vi "Set Property.vi"(0 "Refnum":refnum<vi>, 5 "Colors":refnum<vi>, 7 "Property":T1 {"Mech.Action" items=["Switch when Pressed", "Switch when Released", "Switch until Released", "Latch when Pressed", "Latch when Released", "Latch until Released"]; "Type" items=["Numeric", "Spin Control", "Vertical Slide", "Horizontal Slide", "Push Button", "Rocker", "Vert Rocker", "Horizontal Toggle Switch", "Vertical Toggle Switch", "Slide Switch", "Vertical Slide Switch", "OK Button", "Square Push Button", "Round Push Button", "Vertical Slide Switch2", "Square Push Button2", "Round Push Button2", "Horizontal Slide Switch2", "Round LED", "Square LED"]}, 11 "error in (no error)":errorcluster) -> (15 "error out":errorcluster)   [LabVIEW 2011]
uses:
  Default.ctl
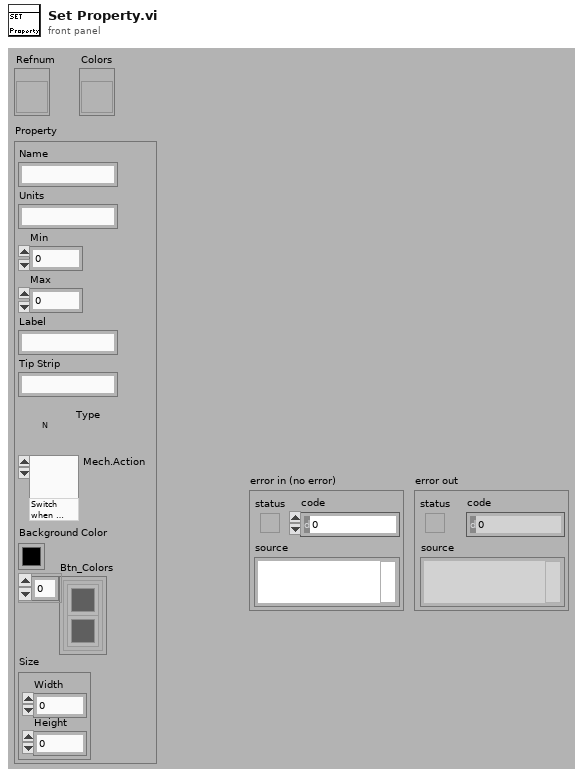
[diagram p1: front panel]
types:
  T1 = typedef "Default.ctl" = cluster{"Name":string, "Units":string, "Min":dbl, "Max":dbl, "Label":string, "Tip Strip":string, "Background Color":u32, "Type":i32, "Mech.Action":u16, "Btn_Colors ":cluster{"FG":u32, "BG":u32}[], "Size":cluster{"Width":u32, "Height":u32}}
  T2 = typedef "LVPositionTypeDef.ctl" = cluster{"Left":i32, "Top":i32}
  T3 = enum8{"Enabled", "Disabled", "Disabled and Grayed Out"}
  T4 = cluster{"Colors [4][0]":cluster{"FG":u32, "BG":u32}, "Colors [4][1]":cluster{"FG":u32, "BG":u32}, "Colors [4][2]":cluster{"FG":u32, "BG":u32}, "Colors [4][3]":cluster{"FG":u32, "BG":u32}}
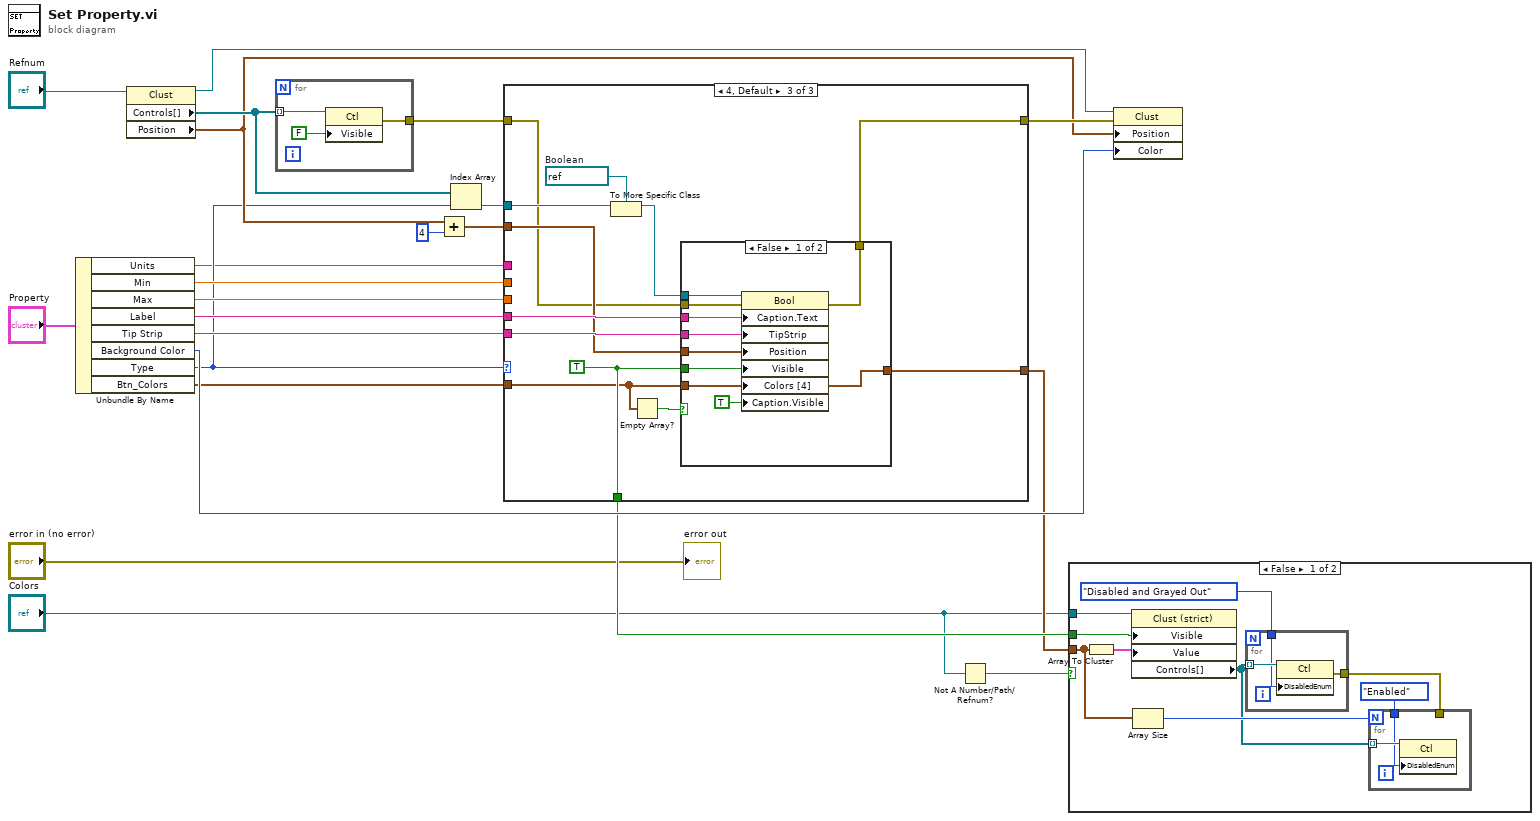
[diagram p0: block diagram]
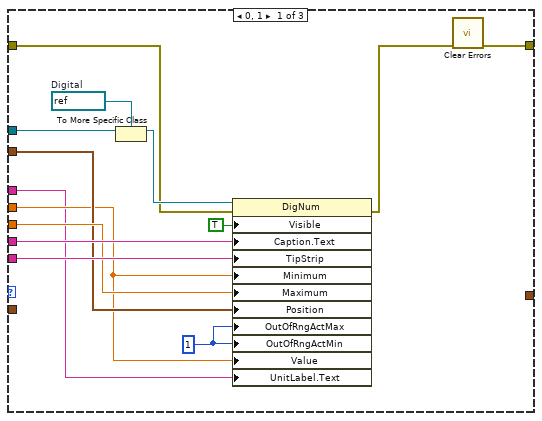
[diagram p3: hidden frame]
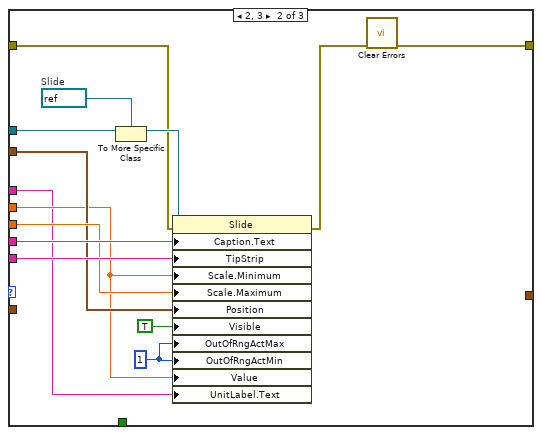
[diagram p4: hidden frame]
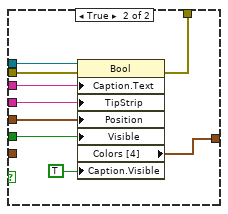
[diagram p5: hidden frame]
diagram:
  n1 = Unbundle By Name("Property") -> ("Units"=w2:string, "Min"=w22:dbl, "Max"=w21:dbl, "Label"=w20:string, "Tip Strip"=w19:string, "Background Color"=w10:u32, "Type"=w9:i32, "Btn_Colors"=w7:cluster{"FG":u32, "BG":u32}[])
  n2 = property class="Clust"(reference="Refnum") -> (reference out=w12:refnum<vi>, "Controls[]"=w17:refnum<vi>[], "Position"=w11:T2)  [unwired: 1 in, 1 out]
  n3 = for {
    tunnel: w17 -> [w26] mode=indexing
    tunnel: [w24] -> w14
    n4 = property class="Ctl"(reference=w26, "Visible"=FALSE) -> (error out=w24:errorcluster)  [unwired: 1 in, 1 out]
  }
  n5 = Add(x=w11, y=4) -> (x+y=w15:T2)
  n6 = Index Array(array=w17, index=w9) -> (element=w16:refnum<vi>)
  n7 = case shown="4, Default" w9 {
    tunnel: w2 -> [w27 w42 _]
    tunnel: w22 -> [w30 w43 _]
    tunnel: w21 -> [w36 w51 _]
    tunnel: w20 -> [w40 w54 w65]
    tunnel: w19 -> [w37 w52 w62]
    tunnel: w16 -> [w35 w50 w66]
    tunnel: w15 -> [w34 w47 w61]
    tunnel: w14 -> [w33 w46 w60]
    tunnel: [w29 w41 w59] -> w13
    tunnel: [_ _ w58] -> w8
    tunnel: w7 -> [_ _ w57]
    tunnel: [_ _ w55] -> w6
    frame 0, 1 {
      w31 = u8 1 ("Response to Value Outside Limits:Maximum")
      w38 = refnum<vi> refnum  # Digital
      n8 = To More Specific Class(target class=w38, reference=w35) -> (specific class reference=w39:refnum<vi>)  [unwired: 1 in, 1 out]
      n9 = property class="DigNum"(reference=w39, error in=w33, "Visible"=TRUE, "Caption.Text"=w40, "TipStrip"=w37, "Minimum"=w30, "Maximum"=w36, "Position"=w34, "OutOfRngActMax"=w31, "OutOfRngActMin"=w31, "Value"=w30, "UnitLabel.Text"=w27) -> (error out=w32:errorcluster)  [unwired: 1 out]
      n10 = call <vilib>:"Clear Errors.vi"("error in (no error)"=w32) -> ("error out"=w29:errorcluster)  [unwired: 6 in]
    }
    frame 2, 3 {
      w44 = u8 1 ("Response to Value Outside Limits:Maximum")
      w49 = refnum<vi> refnum  # Slide
      n11 = To More Specific Class(target class=w49, reference=w50) -> (specific class reference=w53:refnum<vi>)  [unwired: 1 in, 1 out]
      n12 = property class="Slide"(reference=w53, error in=w46, "Caption.Text"=w54, "TipStrip"=w52, "Scale.Minimum"=w43, "Scale.Maximum"=w51, "Position"=w47, "Visible"=TRUE, "OutOfRngActMax"=w44, "OutOfRngActMin"=w44, "Value"=w43, "UnitLabel.Text"=w42) -> (error out=w45:errorcluster)  [unwired: 1 out]
      n13 = call <vilib>:"Clear Errors.vi"("error in (no error)"=w45) -> ("error out"=w41:errorcluster)  [unwired: 6 in]
    }
    frame 4, Default {
      w58 = TRUE ("Visible")
      w63 = refnum<vi> refnum  # Boolean
      n14 = To More Specific Class(target class=w63, reference=w66) -> (specific class reference=w64:refnum<vi>)  [unwired: 1 in, 1 out]
      n15 = Empty Array?(array=w57) -> (empty?=w56:bool)
      n16 = case shown="False" w56 {
        tunnel: w65 -> [w75 w84]
        tunnel: w64 -> [w74 w83]
        tunnel: w62 -> [w73 w82]
        tunnel: w61 -> [w72 w81]
        tunnel: w60 -> [w71 w80]
        tunnel: [w70 w79] -> w59
        tunnel: w58 -> [w69 w78]
        tunnel: w57 -> [w68 _]
        tunnel: [w68 w77] -> w55
        frame False {
          n17 = property class="Bool"(reference=w74, error in=w71, "Caption.Text"=w75, "TipStrip"=w73, "Position"=w72, "Visible"=w69, "Colors [4]"=w68, "Caption.Visible"=TRUE) -> (error out=w70:errorcluster)  [unwired: 1 out]
        }
        frame True {
          n18 = property class="Bool"(reference=w83, error in=w80, "Caption.Text"=w84, "TipStrip"=w82, "Position"=w81, "Visible"=w78, "Caption.Visible"=TRUE) -> (error out=w79:errorcluster, "Colors [4]"=w77:cluster{u32, u32}[])  [unwired: 1 out]
        }
      }
    }
  }
  n19 = Not A Number/Path/Refnum?(number/path/refnum="Colors") -> (NaN/Path/Refnum?=w4:bool)
  n20 = case shown="False" w4 {
    tunnel: w8 -> [w93 _]
    tunnel: w6 -> [w90 _]
    tunnel: "Colors" -> [w92 _]
    frame False {
      n21 = Array To Cluster(array=w90) -> (cluster=w91:T4)
      n22 = property class="Clust (strict)"(reference=w92, "Visible"=w93, "Value"=w91) -> ("Controls[]"=w86:refnum<vi>[])  [unwired: 1 in, 2 out]
      n23 = Array Size(array=w90) -> (size(s)=w88:i32)
      n24 = for {
        tunnel: w86 -> [w98] mode=indexing
        tunnel: T3."Disabled and Grayed Out" ("Disabled") -> [w97]
        tunnel: [w96] -> w85
        n25 = property class="Ctl"(reference=w98, "DisabledEnum"=w97) -> (error out=w96:errorcluster)  [unwired: 1 in, 1 out]
      }
      n26 = for {
        N: w88 -> [_]
        tunnel: w86 -> [w95] mode=indexing
        tunnel: T3."Enabled" ("Disabled") -> [w94]
        tunnel: w85 -> [_]
        n27 = property class="Ctl"(reference=w95, "DisabledEnum"=w94) -> ()  [unwired: 1 in, 2 out]
      }
    }
    frame True {
    }
  }
  n28 = property class="Clust"(reference=w12, error in=w13, "Position"=w11, "Color"=w10) -> ()  [unwired: 2 out]
  "error out" <- "error in (no error)"
